vi "Parse Checksum.vi"(1 "bytes 5 - 101":string="2.7-09 2.7-09 2.7-09 2.7-09 1.0+03 1.0+03 2.5-02 E11m   I5.0-07 P1.0-02 C2.0+00 Q1.0+00 19.1 EDED") -> (0 "checksum":u16 format="%x")   [LabVIEW 2019, in "PGC2D.lvlib"]
uses:
  PGC2D.lvlib
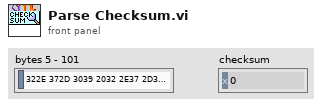
[diagram p1: front panel]
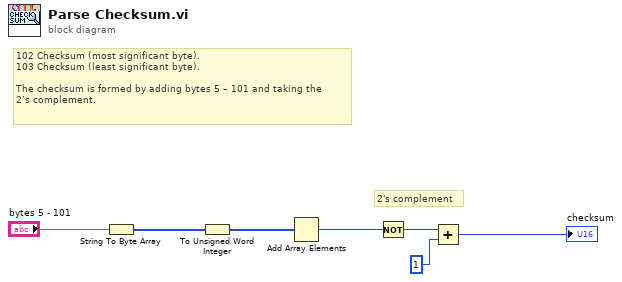
[diagram p0: block diagram]
diagram:
  # "2's complement"
  # "102 Checksum (most significant byte).\n103 Checksum (least significant byte).\n\nThe checksum is formed by adding bytes 5 – 101 and taking the\n2’s complement."
  n1 = String To Byte Array(string="bytes 5 - 101") -> (unsigned byte array=w1:u8[])
  n2 = To Unsigned Word Integer(number=w1) -> (unsigned 16bit integer=w3:u16[])
  n3 = Add Array Elements(numeric array=w3) -> (sum=w5:u16)
  n4 = Not(x=w5) -> (.not. x?=w6:u16)
  n5 = Add(x=w6, y=u16 1) -> (x+y=→"checksum":u16)
